vi "List_All_Object_Types.vi"() -> ()   [LabVIEW 2025]
uses:
  <vilib>/_script/All Supported PropertiesOrMethods TypeDefs/ASC_ArrayOfUniqueIDStringParentIDStringName.ctl
  <vilib>/_script/All Supported PropertiesOrMethods TypeDefs/ASC_UniqueIDStringParentIDStringName.ctl
panel:
  in  "All Types[]":T1
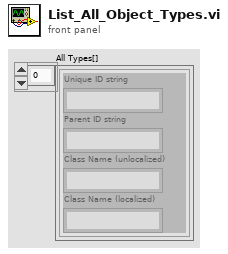
[diagram p1: front panel]
types:
  T1 = typedef "ASC_ArrayOfUniqueIDStringParentIDStringName.ctl" = T2[]
  T2 = typedef "ASC_UniqueIDStringParentIDStringName.ctl" = cluster{"Unique ID string":string, "Parent ID string":string, "Class Name (unlocalized)":string, "Class Name (localized)":string}
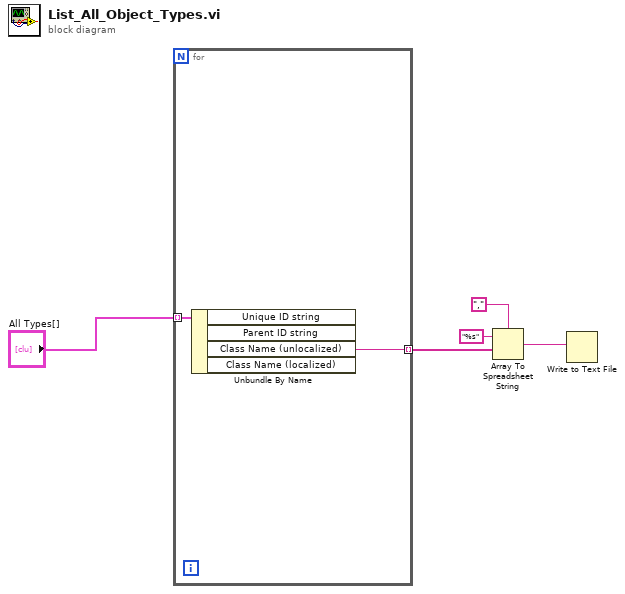
[diagram p0: block diagram]
diagram:
  n1 = for {
    tunnel: "All Types[]" -> [w7] mode=indexing
    tunnel: [w6] -> w5 mode=indexing
    n2 = Unbundle By Name(w7) -> ("Class Name (unlocalized)"=w6:string)  [unwired: 3 out]
  }
  n3 = Array To Spreadsheet String(delimiter (Tab)=",", array=w5, 3:"%s" ("format string")) -> (spreadsheet string=w2:string)
  n4 = Write to Text File(text=w2) -> ()  [unwired: 3 in, 3 out]
